vi "Pueba Daq Elmin y Lester.vi"() -> ()   [LabVIEW 2011]
panel:
  out "encendido":bool
  in  "stop":bool
  out "Alarma de temp.":bool
  out "Meter":i32(knob) scale=0.0..5.0
  out "Cuarta":bool
  out "Tercera":bool
  out "Segunda":bool
  out "Primera":bool
  out "Brake":bool
  out "Acelerar":bool
  out "Velocidad":i32(knob) scale=0.0..220.0
  # "Se tiene que generar la temp del auto de acuerdo a la \nvelocidad:\n1-70 temp 1-2\n70-130 temp 1-4\n130- temp 1-5\nEsto es una entrada que se escribe en la temperatura\ny salida analogica que se ingresa del valor de la temp\nde la DAQ.\n\nEl acelerador cada vez que se pulsa el boton que sera\nuna entrada de la DAQ aumenta la velocidad en 10.\nSi se presiona el boton de brake se rebaja la velocidad en 5.\n\nDebera producirse 4 salidas digitales para representar\ncada uno de los cambios usando led\n1-30 primera\n31-50 segunda\n51-80 tercera\n80- cuarta\n\nLa alarma de la temperatura se enciende solo si esta sube\nde 3 enciende un led en la DAQ, ;a que es una salida\ndigital."
  # "Elmin mejia 21241028"
  # "Lester Roche 21241041"
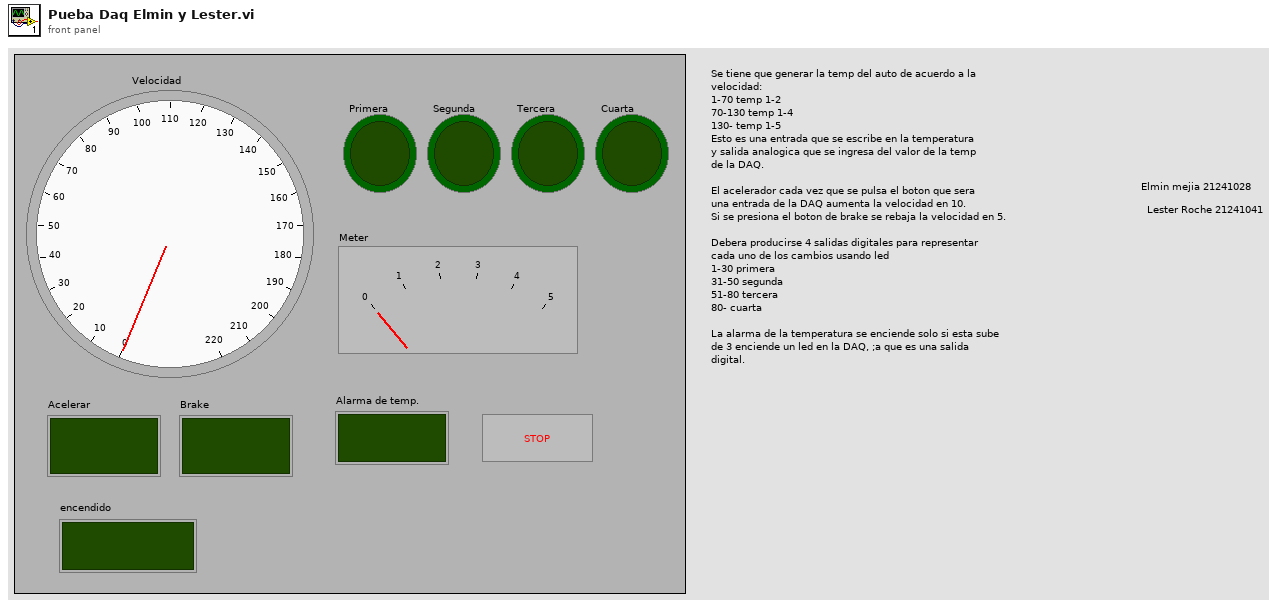
[diagram p1: front panel]
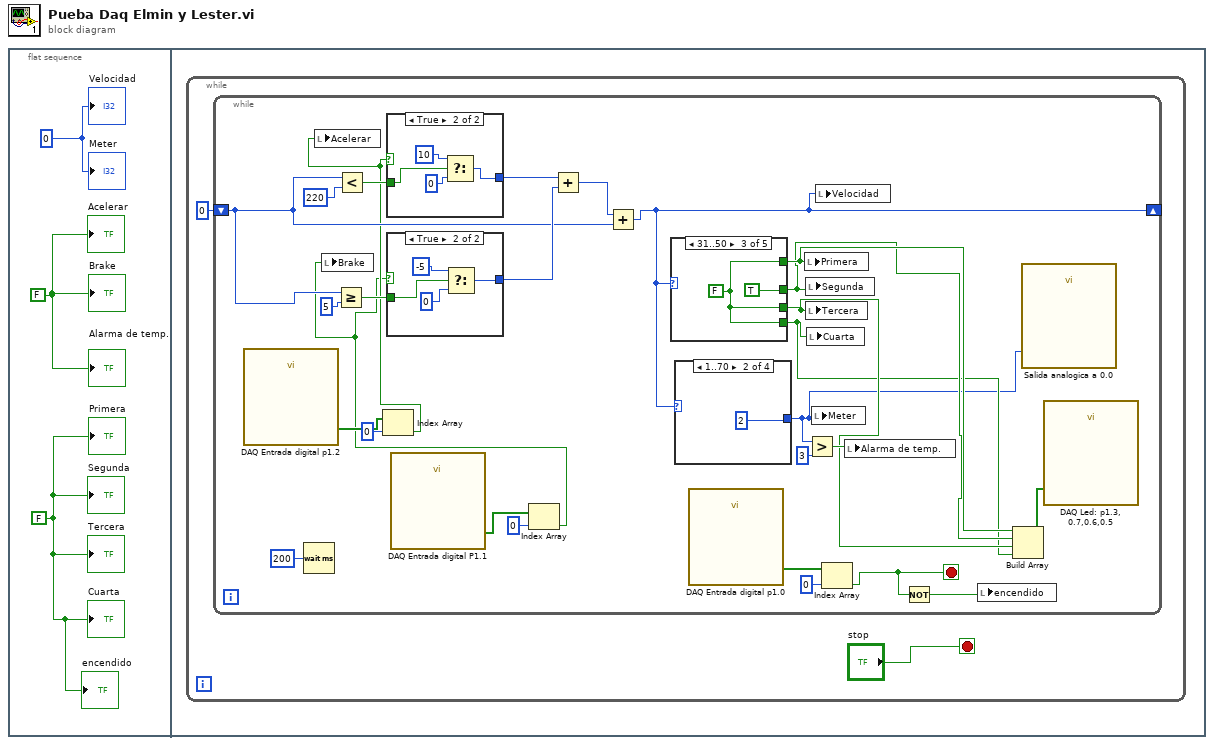
[diagram p0: block diagram]
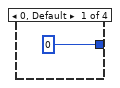
[diagram p2: hidden frame]
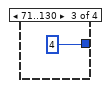
[diagram p3: hidden frame]
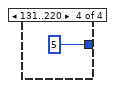
[diagram p4: hidden frame]
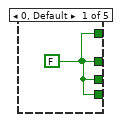
[diagram p5: hidden frame]
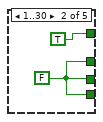
[diagram p6: hidden frame]
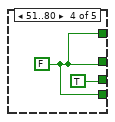
[diagram p7: hidden frame]
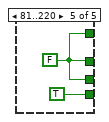
[diagram p8: hidden frame]
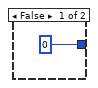
[diagram p9: hidden frame]
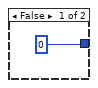
[diagram p10: hidden frame]
diagram:
  n1 = flat-sequence {
    frame #0 {
      w1 = FALSE
      w2 = FALSE
      w3 = 0
      "Velocidad" <- w3
      "Meter" <- w3
      "Acelerar" <- w2
      "Brake" <- w2
      "Alarma de temp." <- w2
      "Primera" <- w1
      "Segunda" <- w1
      "Tercera" <- w1
      "Cuarta" <- w1
      "encendido" <- w1
    }
    frame #1 {
      n2 = while {
        stop <- "stop" stop-if-true
        n3 = while {
          shift-right: [w25] -> _
          shift-left: 0 -> [w26]
          stop <- w7 stop-if-true
          n4 = call "DAQ Entrada digital p1.2"() -> ("data"=w21:bool[])  [unwired: 17 in, 2 out]
          n5 = Wait (ms)(milliseconds to wait=u32 200) -> ()  [unwired: 1 out]
          n6 = Greater Or Equal?(x=w26, y=5) -> (x >= y?=w29:bool)
          n7 = Less?(x=w26, y=220) -> (x < y?=w32:bool)
          n8 = Index Array(array=w21, index=0) -> (element=w19:bool)
          n9 = local write "Acelerar"(w19) -> ()
          n10 = case shown="True" w19 {
            tunnel: w32 -> [_ w56]
            tunnel: [0 w53] -> w31
            frame False {
            }
            frame True {
              n11 = Select(t=10, s=w56, f=0) -> (s? t:f=w53:i32)
            }
          }
          n12 = call "DAQ Entrada digital P1.1"() -> ("data"=w18:bool[])  [unwired: 17 in, 2 out]
          n13 = Index Array(array=w18, index=0) -> (element=w16:bool)
          n14 = local write "Brake"(w16) -> ()
          n15 = case shown="True" w16 {
            tunnel: w29 -> [_ w49]
            tunnel: [0 w48] -> w28
            frame False {
            }
            frame True {
              n16 = Select(t=-5, s=w49, f=0) -> (s? t:f=w48:i32)
            }
          }
          n17 = Add(x=w31, y=w28) -> (x+y=w27:i32)
          n18 = Add(x=w27, y=w26) -> (x+y=w25:i32)
          n19 = case shown="31..50" w25 {
            tunnel: [w38 w39 TRUE w43 w46] -> w14
            tunnel: [w38 TRUE w41 w43 w46] -> w15
            tunnel: [w38 w39 w41 w43 TRUE] -> w12
            tunnel: [w38 w39 w41 TRUE w46] -> w13
            frame 0, Default {
              w38 = FALSE
            }
            frame 1..30 {
              w39 = FALSE
            }
            frame 31..50 {
              w41 = FALSE
            }
            frame 51..80 {
              w43 = FALSE
            }
            frame 81..220 {
              w46 = FALSE
            }
          }
          n20 = case shown="1..70" w25 {
            tunnel: [0 2 4 5] -> w8
            frame 0, Default {
            }
            frame 1..70 {
            }
            frame 71..130 {
            }
            frame 131..220 {
            }
          }
          n21 = call "DAQ Entrada digital p1.0"() -> ("data"=w10:bool[])  [unwired: 17 in, 2 out]
          n22 = local write "Primera"(w15) -> ()
          n23 = local write "Segunda"(w14) -> ()
          n24 = local write "Tercera"(w13) -> ()
          n25 = local write "Cuarta"(w12) -> ()
          n26 = Greater?(x=w8, y=3) -> (0:w22:bool)
          n27 = local write "Meter"(w8) -> ()
          n28 = local write "Velocidad"(w25) -> ()
          n29 = Index Array(array=w10, index=0) -> (element=w7:bool)
          n30 = local write "Alarma de temp."(w22) -> ()
          n31 = Not(x=w7) -> (.not. x?=w6:bool)
          n32 = local write "encendido"(w6) -> ()
          n33 = Build Array(w15, w14, w13, w12) -> (w11:bool[])
          n34 = call "Salida analogica a 0.0"("data"=w8) -> ()  [unwired: 17 in, 2 out]
          n35 = call "DAQ Led: p1.3, 0.7,0.6,0.5"("data"=w11) -> ()  [unwired: 17 in, 2 out]
        }
      }
    }
  }
